vi "Simulate Temperature Acquisition - Station 3.vi"() -> (3 "Temperature":dbl)   [LabVIEW 2019]
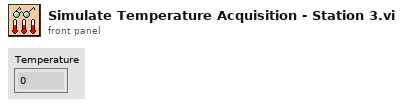
[diagram p1: front panel]
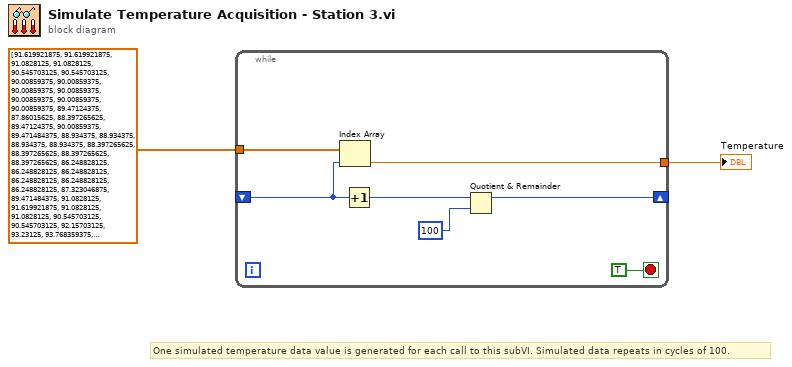
[diagram p0: block diagram]
diagram:
  # "One simulated temperature data value is generated for each call to this subVI. Simulated data repeats in cycles of 100."
  n1 = while {
    tunnel: dbl[] [91.619921875, 91.619921875, 91.0828125, 91.0828125, 90.545703125, 90.545703125, 90.00859375, 90.00859375, 90.00859375, 90.00859375, 90.00859375, 90.00859375, 90.00859375, 89.47124375, 87.86015625, 88.397265625, 89.47124375, 90.00859375, 89.471484375, 88.934375, 88.934375, 88.934375, 88.934375, 88.397265625, 88.397265625, 88.397265625, 88.397265625, 86.248828125, 86.248828125, 86.248828125, 86.248828125, 86.248828125, 86.248828125, 87.323046875, 89.471484375, 91.0828125, 91.619921875, 91.0828125, 91.0828125, 90.545703125, 90.545703125, 92.15703125, 93.23125, 93.768359375, 94.30546875, 94.30546875, 94.842578125, 94.30546875, 93.768359375, 93.23125, 92.694140625, 92.694140625, 92.15703125, 91.619921875, 91.0828125, 91.0828125, 91.0828125, 91.0828125, 91.0828125, 90.545703125, 90.545703125, 90.00859375, 90.00859375, 90.00859375, 91.0828125, 91.619921875, 92.15703125, 92.694140625, 93.768359375, 94.30546875, 94.30546875, 94.30546875, 93.768359375, 93.23125, 92.694140625, 93.23125, 94.30546875, 94.842578125, 95.3796875, 94.842578125, 94.30546875, 94.30546875, 93.23125, 93.23125, 93.23125, 92.15703125, 92.15703125, 92.15703125, 91.619921875, 91.619921875, 92.694140625, 93.23125, 94.30546875, 94.30546875, 93.768359375, 93.23125, 92.694140625, 92.694140625, 92.15703125, 92.15703125] ("array w/ subset deleted") -> [w8]
    tunnel: [w7] -> w2
    shift-right: [w5] -> _
    shift-left: _ -> [w3]
    stop <- TRUE stop-if-true
    n2 = Index Array(array=w8, index=w3) -> (element=w7:dbl)
    n3 = Increment(x=w3) -> (x+1=w4:i32)
    n4 = Quotient & Remainder(x=w4, y=100) -> (x-y*floor(x/y)=w5:i32)  [unwired: 1 out]
  }
  "Temperature" <- w2
